vi "InitializeFPGA.vi"() -> (0 "error out":errorcluster, 1 "FPGA VI Reference Out":refnum<k20>)   [LabVIEW 2016]
uses:
  <vilib>/FPGAPlugInAG/cRIO-9033/niLvFpga_Open_cRIO-9033.vi
  Instance           2 22Saved   InitializeFPGA .vi
  <vilib>/rvi/interface/nirviOpenFPGA/nirviOpenFPGA.xnode
  FPGA Bitfiles/EV-MCU_FPGATarget_CANEngine(FPGA)b_eM8Xz3qYJVA.lvbitx
  CAN_Engine(FPGA)_basic.vi
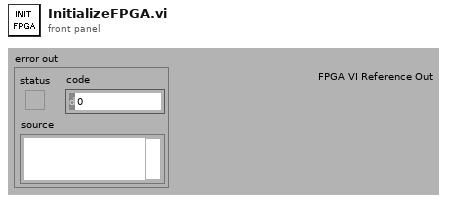
[diagram p1: front panel]
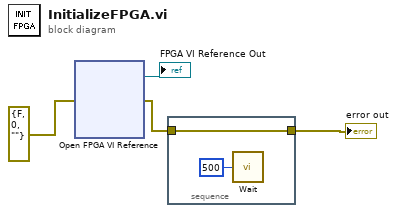
[diagram p0: block diagram]
diagram:
  n1 = xnode "Open FPGA VI Reference"("error in"=errorcluster {"status"=FALSE, "code"=0, "source"=""}) -> ("FPGA VI Reference Out"=→"FPGA VI Reference Out":refnum<k20>, "error out"=w3:errorcluster)  [unwired: 1 in]
  n2 = stacked-sequence {
    tunnel: w3 -> [w6]
    tunnel: [w6] -> w4
    frame #0 {
      n3 = call "Wait"("Count(mSec)"=u32 500) -> ()  [unwired: 1 out]
    }
  }
  "error out" <- w4
